vi "Unflatten.vi"(8 "error in (no error)":errorcluster, 9 "timeout in":bool, 10 "Data In":refnum<data-value>[](array[refnum]), 11 "CIFFifoCAN in":refnum<class "CIF_NIChn_Fifo_DAQ.lvclass">) -> (0 "error out":errorcluster, 2 "Data Out":refnum<data-value>[](array[refnum]), 3 "CIFFifoCAN out":refnum<class "CIF_NIChn_Fifo_DAQ.lvclass">, 4 "Header":T1)   [LabVIEW 2021, in "CIF_NIChn_Fifo_DAQ.lvclass"]
uses:
  CIF_NIChn_Fifo_DAQ.lvclass
  ChannelCommon/typedef/FIFO Header.ctl
  ChannelCommon/ChannelCommon.lvlib
  ChannelCommon/typedef/Datatype Waveform.ctl
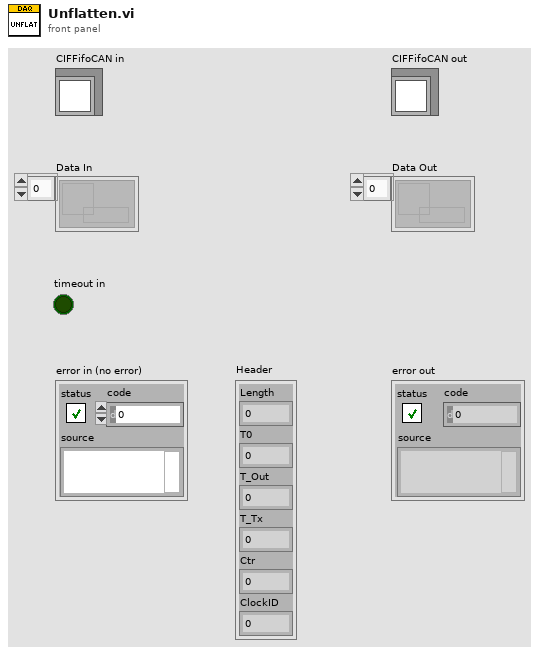
[diagram p1: front panel]
types:
  T1 = typedef "ChannelCommon.lvlib/FIFO Header.ctl" = cluster{"Length":u64, "T0":i64, "T_Out":i64, "T_Tx":i64, "Ctr":u64, "ClockID":u8}
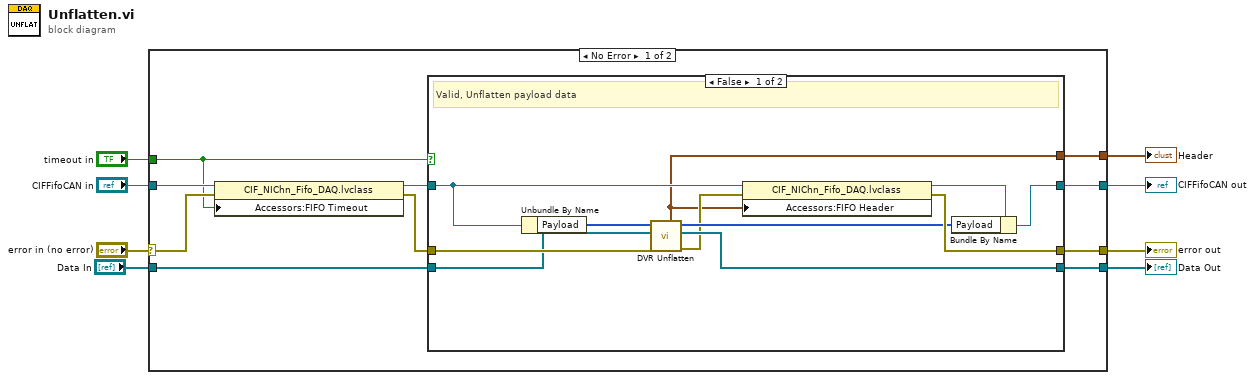
[diagram p0: block diagram]
diagram:
  n1 = case shown="No Error" "error in (no error)" {
    selector: "error in (no error)" -> [w10 w34]
    tunnel: [w15 w34] -> w7
    tunnel: [w16 w33] -> w5
    tunnel: "CIFFifoCAN in" -> [w13 w33]
    tunnel: "timeout in" -> [w9 _]
    tunnel: [w18 _] -> w2
    tunnel: [w17 _] -> w3
    tunnel: "Data In" -> [w14 _]
    frame No Error {
      n2 = property class="CIF_NIChn_Fifo_DAQ.lvclass"(reference=w13, error in=w10, "Accessors:FIFO Timeout"=w9) -> (reference out=w12:refnum<class "CIF_NIChn_Fifo_DAQ.lvclass">, error out=w11:errorcluster)
      n3 = case shown="False" w9 {
        tunnel: w11 -> [w29 w31]
        tunnel: w12 -> [w21 w32]
        tunnel: [w28 w30] -> w18
        tunnel: [w20 _] -> w17
        tunnel: [w27 w32] -> w16
        tunnel: [w26 w31] -> w15
        tunnel: w14 -> [w25 w30]
        frame False {
          # "Valid, Unflatten payload data"
          n4 = Unbundle By Name(w21) -> ("Payload"=w23:u8[])
          n5 = call "DVR Unflatten.vi"("error in (no error)"=w29, "DVRs In"=w25, "Flatten Data in"=w23) -> ("error out"=w22:errorcluster, "DVRs Out"=w28:refnum<data-value>[], "Flatten Data out"=w24:u8[], "Header out"=w20:T1)  [unwired: 5 in]
          n6 = property class="CIF_NIChn_Fifo_DAQ.lvclass"(reference=w21, error in=w22, "Accessors:FIFO Header"=w20) -> (reference out=w19:refnum<class "CIF_NIChn_Fifo_DAQ.lvclass">, error out=w26:errorcluster)
          n7 = Bundle By Name(cluster=w19, "Payload"=w24) -> (w27:refnum<class "CIF_NIChn_Fifo_DAQ.lvclass">)
        }
        frame True {
          # "Timeout"
        }
      }
    }
    frame Error {
    }
  }
  "error out" <- w7
  "CIFFifoCAN out" <- w5
  "Header" <- w3
  "Data Out" <- w2
